vi "CreateElement.vi"(8 "error in":errorcluster, 11 "Document in":refnum<k20>) -> (0 "error out":errorcluster, 2 "Element":refnum<k20>, 3 "Document out":refnum<k20>)   [LabVIEW 2021, in "ProligentXMLGenerator.lvlib" / "Datawarehouse.lvclass"]
uses:
  Datawarehouse.lvclass
  Datawarehouse.lvclass/Datawarehouse.ctl
  <resource>/objmgr/DOMUserDefRef.rc
  <vilib>/xml/NI_XML.lvlib
  Base/DOMSupport/DOMSupport.lvlib
  <vilib>/xml/Close Reference(Node).vi
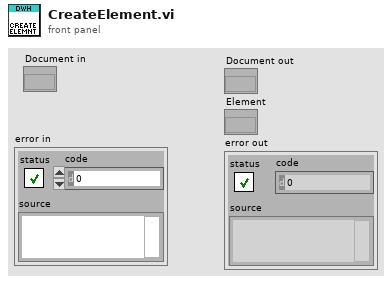
[diagram p1: front panel]
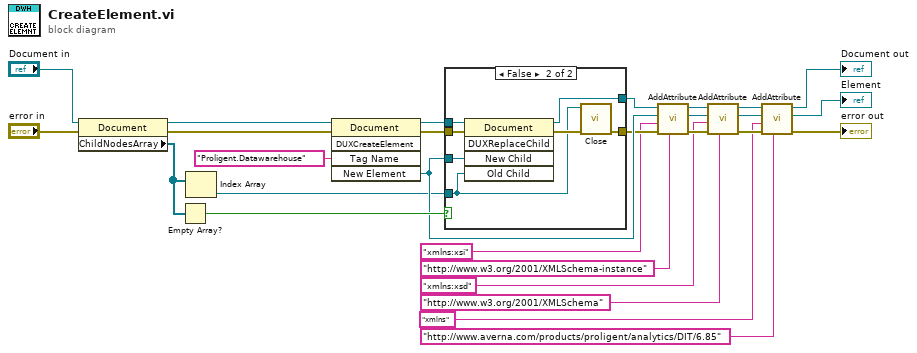
[diagram p0: block diagram]
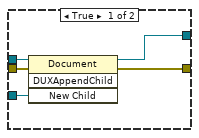
[diagram p2: hidden frame]
diagram:
  n1 = property on="Property Node" class="Document"(reference="Document in", error in="error in") -> (reference out=w24:refnum<k20>, error out=w25:errorcluster, "ChildNodesArray"=w21:refnum<k20>[])
  n2 = Empty Array?(array=w21) -> (empty?=w23:bool)
  n3 = Index Array(array=w21) -> (element=w1:refnum<k20>)  [unwired: 1 in]
  n4 = invoke on="Invoke Node" class="Document" method="DUXCreateElement"(reference=w24, error in=w25, "Tag Name"="Proligent.Datawarehouse") -> (reference out=w27:refnum<k20>, error out=w26:errorcluster, "New Element"=w12:refnum<k20>)  [unwired: 2 in, 2 out]
  n5 = case shown="False" w23 {
    tunnel: w27 -> [w33 w40]
    tunnel: w26 -> [w32 w39]
    tunnel: [w31 w36] -> w8
    tunnel: [w30 w38] -> w17
    tunnel: w12 -> [w29 w37]
    tunnel: w1 -> [_ w34]
    frame True {
      n6 = invoke on="Invoke Node" class="Document" method="DUXAppendChild"(reference=w33, error in=w32, "New Child"=w29) -> (reference out=w30:refnum<k20>, error out=w31:errorcluster)  [unwired: 1 in, 2 out]
    }
    frame False {
      n7 = invoke on="Invoke Node" class="Document" method="DUXReplaceChild"(reference=w40, error in=w39, "New Child"=w37, "Old Child"=w34) -> (reference out=w38:refnum<k20>, error out=w35:errorcluster)  [unwired: 1 in, 3 out]
      n8 = call-poly <vilib>:"Close.vi"("error in (no error)"=w35, "node"=w34) -> ("error out"=w36:errorcluster)  [unwired: 7 in]
    }
  }
  n9 = call "AddAttribute.vi"("Value"="http://www.w3.org/2001/XMLSchema-instance", "error in"=w8, "Name"="xmlns:xsi", "OwningElement in"=w12, "Document in"=w17) -> ("error out"=w19:errorcluster, "OwningElement out"=w13:refnum<k20>, "Document out"=w16:refnum<k20>)  [unwired: 4 in]
  n10 = call "AddAttribute.vi"("Value"="http://www.w3.org/2001/XMLSchema", "error in"=w19, "Name"="xmlns:xsd", "OwningElement in"=w13, "Document in"=w16) -> ("error out"=w18:errorcluster, "OwningElement out"=w14:refnum<k20>, "Document out"=w15:refnum<k20>)  [unwired: 4 in]
  n11 = call "AddAttribute.vi"("Value"="http://www.averna.com/products/proligent/analytics/DIT/6.85", "error in"=w18, "Name"="xmlns", "OwningElement in"=w14, "Document in"=w15) -> ("error out"=→"error out":errorcluster, "OwningElement out"=→"Element":refnum<k20>, "Document out"=→"Document out":refnum<k20>)  [unwired: 4 in]
